vi "ZLockDisconnect.vi"(8 "error in (no error)":errorcluster, 11 "ZLock in":refnum<class "ZLock.lvclass">) -> (0 "error out":errorcluster, 3 "ZLock out":refnum<class "ZLock.lvclass">)   [LabVIEW 2010, in "ZLock.lvclass"]
uses:
  <userlib>/bias/subvis/zlock/ZLock.lvclass
  <userlib>/bias/subvis/zlock/ZLock.lvclass/ZLock.ctl
  <vilib>/addons/zeromq/pointer.ctl
  <vilib>/addons/zeromq/zeromq.lvlib
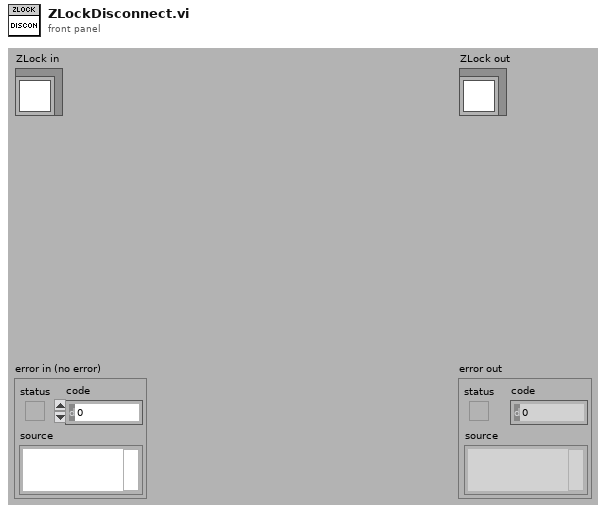
[diagram p1: front panel]
types:
  T1 = typedef "pointer.ctl" = u64
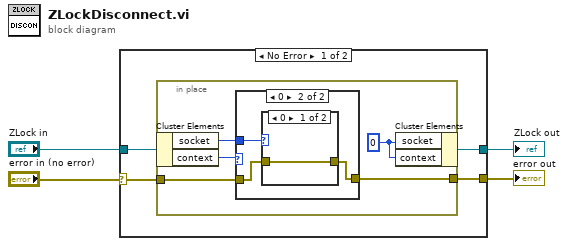
[diagram p0: block diagram]
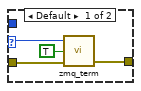
[diagram p2: hidden frame]
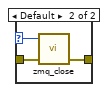
[diagram p3: hidden frame]
diagram:
  n1 = case shown="No Error" "error in (no error)" {
    selector: "error in (no error)" -> [w6 w26]
    tunnel: [w7 w26] -> w3
    tunnel: [w5 w25] -> w1
    tunnel: "ZLock in" -> [w8 w25]
    frame No Error {
      n2 = in-place {
        in-place-border: w6 -> [w11]
        in-place-border: [w10] -> w7
        w9 = T1 0 ("context")
        n3 = in-place-cluster #1(w8) -> ("socket"=w12:T1, "context"=w13:T1)
        n4 = case shown="0" w13 {
          selector: w13 -> [w17 _]
          tunnel: w11 -> [w15 w20]
          tunnel: w12 -> [_ w19]
          tunnel: [w14 w18] -> w10
          frame Default {
            n5 = call <vilib>:"zmq_term.vi"("error in"=w15, "reap? (F)"=TRUE, "context"=w17) -> ("error out"=w14:errorcluster)  [unwired: 2 in]
          }
          frame 0 {
            n6 = case shown="0" w19 {
              selector: w19 -> [_ w23]
              tunnel: w20 -> [w21 w24]
              tunnel: [w21 w22] -> w18
              frame 0 {
              }
              frame Default {
                n7 = call <vilib>:"zmq_close.vi"("error in"=w24, "socket in"=w23) -> ("error out"=w22:errorcluster)  [unwired: 3 in]
              }
            }
          }
        }
        n8 = in-place-cluster #1("socket"=w9, "context"=w9) -> (w5:refnum<class "ZLock.lvclass">)
      }
    }
    frame Error {
    }
  }
  "error out" <- w3
  "ZLock out" <- w1
